vi "Date.vi"() -> (0 "chaîne de date/heure":string)   [LabVIEW 2010]
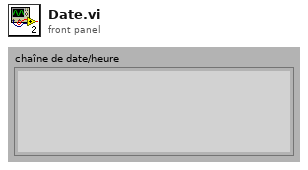
[diagram p1: front panel]
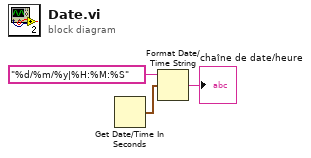
[diagram p0: block diagram]
diagram:
  n1 = Get Date/Time In Seconds() -> (seconds since 1Jan1904=w1:timestamp)
  n2 = Format Date/Time String(time format string (%c)="%d/%m/%y|%H:%M:%S" ("chaîne de format de l'heure (%c)"), seconds (now)=w1) -> (date/time string=→"chaîne de date/heure":string)  [unwired: 1 in]
